vi "Execute.vi"(7 "Actor in":refnum<class "Actor.lvclass">, 8 "Error in":errorcluster, 11 "Stopping Msg in":refnum<class "Stopping Msg.lvclass">) -> (0 "Error out":errorcluster, 2 "Msg Output":refnum<class "Msg Output.lvclass">, 5 "Actor out":refnum<class "Actor.lvclass">)   [LabVIEW 2020, in "jettl.lvlib" / "Stopping jettl Msg.lvlib" / "Stopping Msg.lvlib" / "Stopping Msg.lvclass"]
doc: "jettl 6.12.1.94\nNathan Davis - Nathan Davis\nCopyright (c) 2026, Nathan Davis\nMIT"
uses:
  Stopping Msg.lvclass
  Actor/Actor.lvclass
  Msg Output/Msg Output.lvclass
  Stopping jettl Msg/Stopping jettl Msg.lvclass
  Stopping Msg Output/Stopping Msg Output.lvlib
  Stopping Msg Input/Stopping Msg Input.lvlib
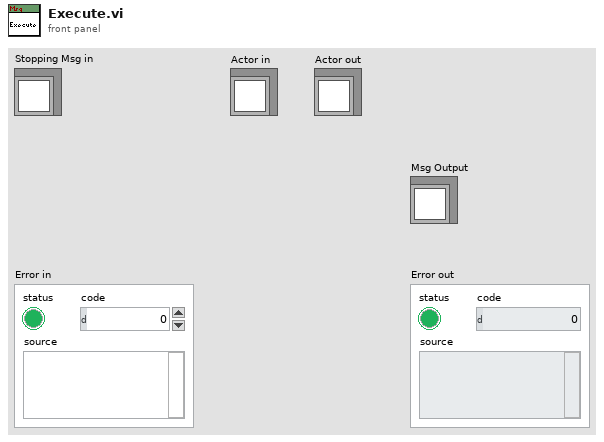
[diagram p1: front panel]
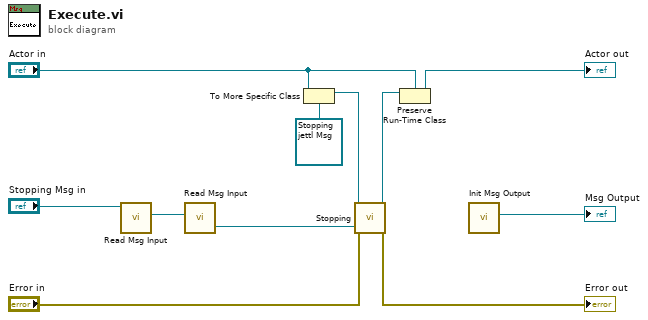
[diagram p0: block diagram]
diagram:
  n1 = call-dynamic "Read Msg Input.vi"("Stopping Msg in"="Stopping Msg in") -> ("Msg Input"=w3:refnum<class "Msg Input.lvclass">)  [unwired: 10 in]
  n2 = call "Read Msg Input.vi"("Msg Input"=w3) -> ("Teller"=w1:refnum<class "Teller.lvclass">)  [unwired: 10 in]
  n3 = To More Specific Class(target class=refnum<class "Stopping jettl Msg.lvclass"> refnum ("jettl Msg Template"), reference="Actor in") -> (specific class reference=w10:refnum<class "Stopping jettl Msg.lvclass">)  [unwired: 1 in, 1 out]
  n4 = call-dynamic "Stopping.vi"("Teller"=w1, "Error in"="Error in", "Stopping jettl Msg in"=w10) -> ("Error out"=→"Error out":errorcluster, "Stopping jettl Msg out"=w9:refnum<class "Stopping jettl Msg.lvclass">)  [unwired: 7 in]
  n5 = Preserve Run-Time Class(object in=w9, 2:"Actor in") -> (object out=→"Actor out":refnum<class "Actor.lvclass">)  [unwired: 1 in, 1 out]
  n6 = call "Init Msg Output.vi"() -> ("Msg Output"=→"Msg Output":refnum<class "Msg Output.lvclass">)  [unwired: 11 in]
